vi "Machine_details_log.vi"(0 "Delete Old data?":bool, 1 "Machine name":string, 2 "Branch Name":string, 3 "error in":errorcluster) -> (4 "Brach Name":string, 5 "Document Path":path, 6 "HTML TEXT":string, 7 "current time":timestamp, 8 "error out":errorcluster)   [LabVIEW 2013]
uses:
  <vilib>/Utility/NIReport.llb/NI_report.lvclass
panel:
  out "Machine name":string
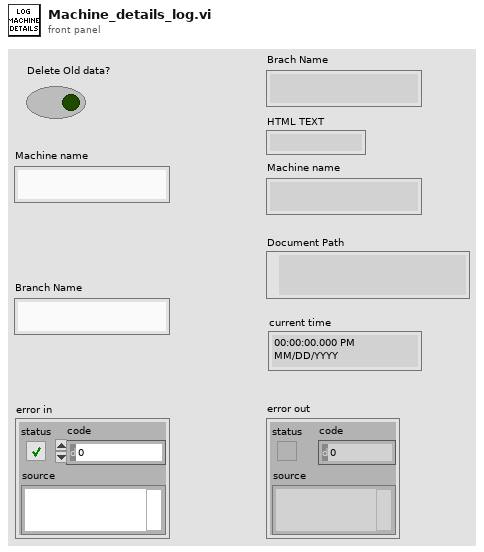
[diagram p1: front panel]
types:
  T1 = enum16{"Standard Report", "HTML", "Word", "Excel"}
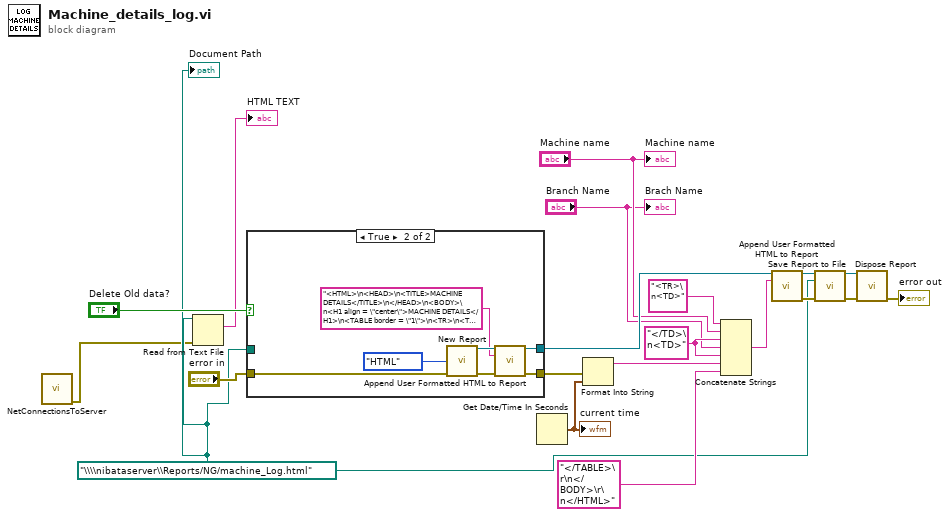
[diagram p0: block diagram]
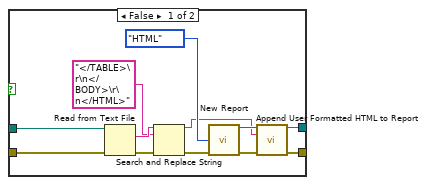
[diagram p2: hidden frame]
diagram:
  w2 = path "\\\\nibataserver\\Reports/NG/machine_Log.html"
  w13 = "</TD>\n<TD>"
  n1 = call "NetConnectionsToServer.vi"() -> ("error out"=w1:errorcluster)  [unwired: 11 in]
  n2 = Read from Text File(file (use dialog)=w2, error in=w1) -> (text=→"HTML TEXT":string)  [unwired: 2 in, 3 out]
  n3 = case shown="True" "Delete Old data?" {
    tunnel: "error in" -> [w24 w38]
    tunnel: w2 -> [w23 _]
    tunnel: [w22 w35] -> w11
    tunnel: [w21 w36] -> w9
    frame False {
      n4 = Read from Text File(file (use dialog)=w23, error in=w24) -> (text=w29:string, error out=w28:errorcluster)  [unwired: 2 in, 2 out]
      n5 = Search and Replace String(input string=w29, search string="</TABLE>\r\n</BODY>\r\n</HTML>", error in=w28) -> (result string=w25:string, error out=w26:errorcluster)  [unwired: 5 in, 2 out]
      n6 = call <vilib>:"New Report.vi"("report type"=T1."HTML", "error in (no error)"=w26) -> ("report out"=w30:refnum<class "NI_report.lvclass">, "error out"=w31:errorcluster)  [unwired: 12 in]
      n7 = call-dynamic "Append User Formatted HTML to Report.vi"("report in"=w30, "HTML text"=w25, "error in (no error)"=w31) -> ("report out"=w22:refnum<class "NI_report.lvclass">, "error out"=w21:errorcluster)  [unwired: 11 in]
    }
    frame True {
      n8 = call <vilib>:"New Report.vi"("report type"=T1."HTML", "error in (no error)"=w38) -> ("report out"=w34:refnum<class "NI_report.lvclass">, "error out"=w37:errorcluster)  [unwired: 12 in]
      n9 = call-dynamic "Append User Formatted HTML to Report.vi"("report in"=w34, "HTML text"="<HTML>\n<HEAD>\n<TITLE>MACHINE DETAILS</TITLE>\n</HEAD>\n<BODY>\n<H1 align = \"center\">MACHINE DETAILS</H1>\n<TABLE border = \"1\">\n<TR>\n<TD align = \"center\"><B> MACHINE </B></TD>\n<TD align = \"center\"><B> BRANCH </B></TD>\n<TD align = \"center\"><B> TIME </B></TD>\n</TR>", "error in (no error)"=w37) -> ("report out"=w35:refnum<class "NI_report.lvclass">, "error out"=w36:errorcluster)  [unwired: 11 in]
    }
  }
  n10 = Get Date/Time In Seconds() -> (seconds since 1Jan1904=w10:timestamp)
  "current time" <- w10
  n11 = Format Into String(error in=w9, w10) -> (resulting string=w14:string)  [unwired: 2 in, 1 out]
  n12 = Concatenate Strings("<TR>\n<TD>", "Machine name", w13, "Branch Name", w13, w14, "</TABLE>\r\n</BODY>\r\n</HTML>") -> (w15:string)
  n13 = call-dynamic "Append User Formatted HTML to Report.vi"("report in"=w11, "HTML text"=w15) -> ("report out"=w17:refnum<class "NI_report.lvclass">, "error out"=w18:errorcluster)  [unwired: 12 in]
  n14 = call-dynamic "Save Report to File.vi"("report in"=w17, "report file path"=w2, "error in (no error)"=w18) -> ("report out"=w7:refnum<class "NI_report.lvclass">, "error out"=w6:errorcluster)  [unwired: 11 in]
  n15 = call-dynamic "Dispose Report.vi"("report in"=w7, "error in (no error)"=w6) -> ("error out"=→"error out":errorcluster)  [unwired: 13 in]
  "Document Path" <- w2
  "Machine name" <- "Machine name"
  "Brach Name" <- "Branch Name"
